vi "Test_Read_Dataset_From_Disk.vi"(8 "error in (no error)":errorcluster) -> (0 "error out":errorcluster)   [LabVIEW 2018]
doc: "This VI inits a waveform generation session for AWG-5421. This is a basic example that shows how to setup the board in order to generate waveforms according to a script. \nBy default this configuration uses one channel CH0, and one script trigger ScriptTrigger0. The ScriptTrigger0 is waiting for an external trigger : i.e. a digital Edge on pin PFI 0 by default.\n\nThere are various options for the script to be used. Consult the Script control help for more information on configuring the example for specific scripts."
uses:
  <vilib>/Analysis/NI_AALPro.lvlib
panel:
  in  "Cut Data ?":bool
  out "Mass Spectrum 2":cluster{"mass":sgl[], sgl[]}(graph)
  out "Mass Spectrum":cluster{"mass":sgl[], sgl[]}(graph)
  out "Signal 2":cluster{sgl[], sgl[]}(graph)
  out "df 2":dbl caption="df" format="%0.2f"
  out "Frequency Spectrum 2":cluster{dbl[], dbl[]}(graph)
  in  "End Signal":i32=200000
  in  "Start Signal":i32
  out "offset":sgl
  out "Frequency Spectrum":cluster{dbl[], "Power Spectrum (V^2 rms)":dbl[]}(graph)
  out "df":dbl format="%0.2f"
  out "Vertical Range in data":sgl
  out "Signal":cluster{sgl[], sgl[]}(graph)
  out "Time Step":sgl
  in  "chemin du fichier":path=path "D:/PIRENEA/DATA/2016/data_2016_11_22/2016_11_22_016.A00"
  out "Data Size (samples)":i32
  out "Total Size (bytes)":i64
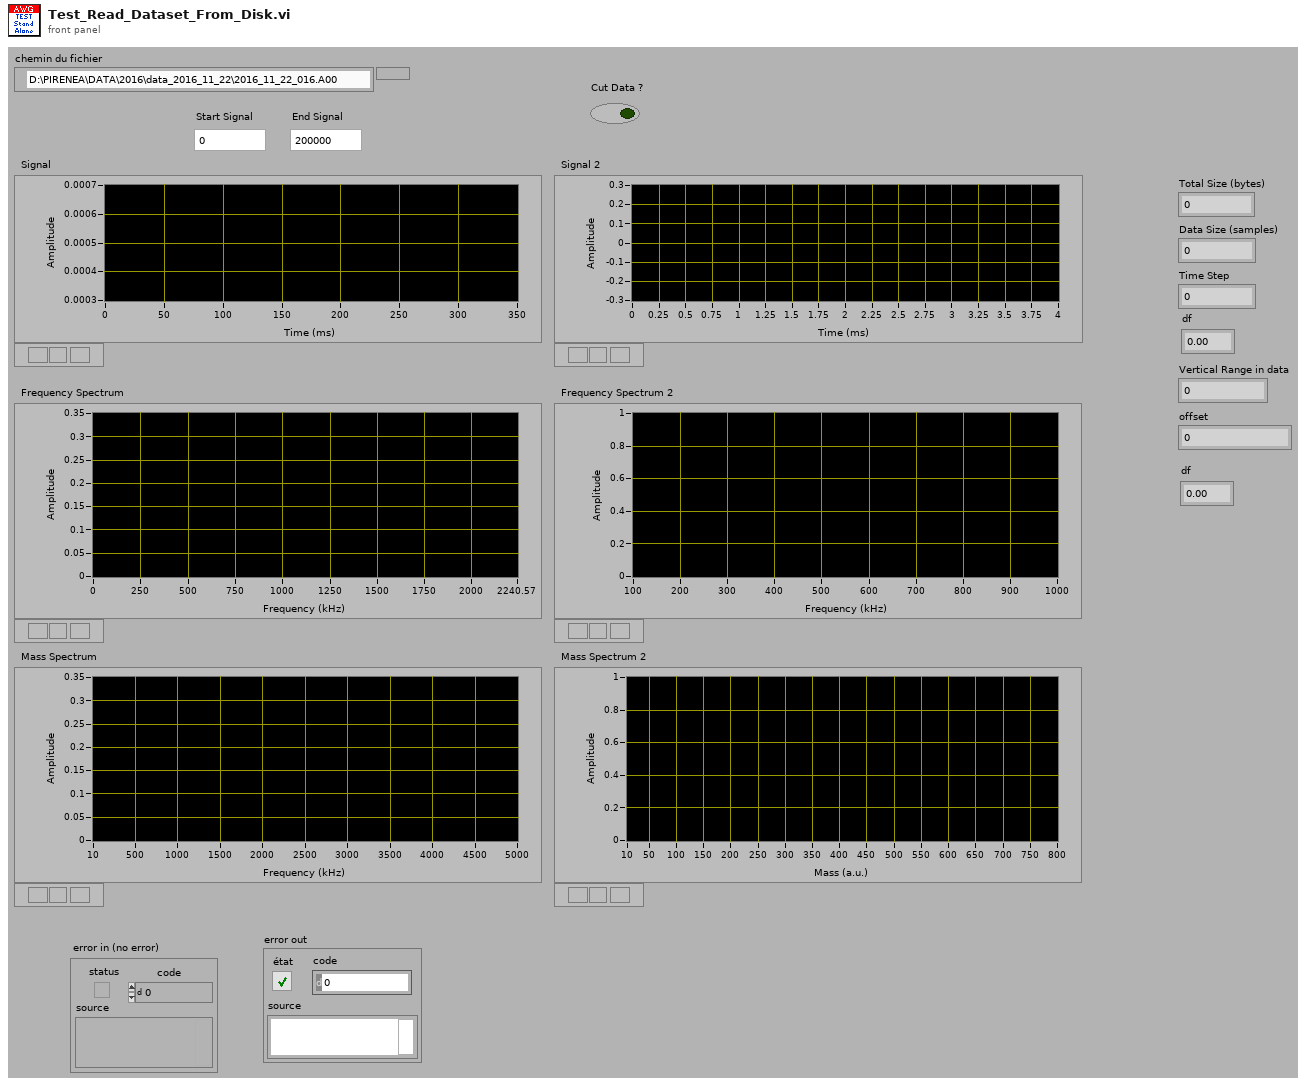
[diagram p1: front panel]
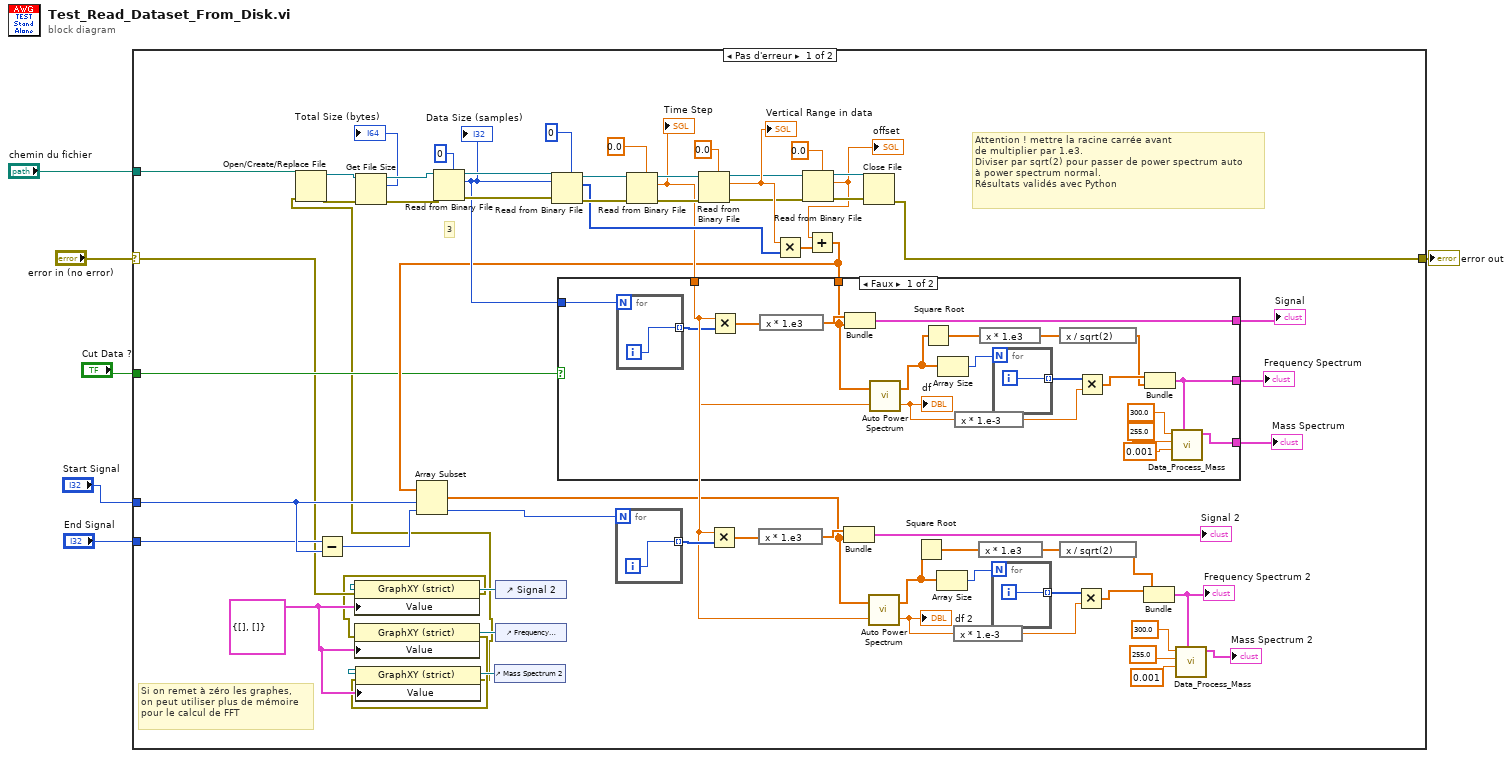
[diagram p0: block diagram]
diagram:
  n1 = case shown="Pas d'erreur" "error in (no error)" {
    selector: "error in (no error)" -> [w10 w95]
    tunnel: [w53 w95] -> w6
    tunnel: "chemin du fichier" -> [w60 _]
    tunnel: "Start Signal" -> [w24 _]
    tunnel: "End Signal" -> [w23 _]
    tunnel: "Cut Data ?" -> [w18 _]
    frame No Error {
      w11 = cluster{sgl[], sgl[]} {[], []} ("Valeur")
      # "Si on remet à zéro les graphes,\non peut utiliser plus de mémoire\npour le calcul de FFT"
      # "Attention ! mettre la racine carrée avant\nde multiplier par 1.e3.\nDiviser par sqrt(2) pour passer de power spectrum auto\nà power spectrum normal.\nRésultats validés avec Python"
      # "3"
      n2 = Subtract(x=w23, y=w24) -> (x-y=w32:i32)
      n3 = control-ref of="Mass Spectrum 2"() -> (w12:refnum<vi>)
      n4 = control-ref of="Signal 2"() -> (w14:refnum<vi>)
      n5 = property class="GraphXY (strict)"(reference=w14, error in=w10, "Value"=w11) -> (error out=w9:errorcluster)  [unwired: 1 out]
      n6 = control-ref of="Frequency Spectrum 2"() -> (w13:refnum<vi>)
      n7 = property class="GraphXY (strict)"(reference=w13, error in=w9, "Value"=w11) -> (error out=w8:errorcluster)  [unwired: 1 out]
      n8 = property class="GraphXY (strict)"(reference=w12, error in=w8, "Value"=w11) -> (error out=w7:errorcluster)  [unwired: 1 out]
      n9 = Open/Create/Replace File(file path (use dialog)=w60, error in=w7) -> (refnum out=w68:refnum<file>, error out=w67:errorcluster)  [unwired: 4 in, 1 out]
      n10 = Get File Size(file=w68, error in=w67) -> (refnum out=w66:refnum<file>, size (in bytes)=→"Total Size (bytes)":i64, 0:w65:errorcluster)
      n11 = Read from Binary File(5:0, 8:w65, 11:w66) -> (0:w62:errorcluster, 2:w51:i32, 3:w63:refnum<file>)  [unwired: 3 in, 1 out]
      "Data Size (samples)" <- w51
      n12 = Read from Binary File(5:i16 0, 8:w62, 10:w51, 11:w63) -> (0:w58:errorcluster, 2:w52:i16[], 3:w59:refnum<file>)  [unwired: 2 in, 1 out]
      n13 = for {
        N: w32 -> [_]
        tunnel: [w94] -> w33 mode=indexing
        i -> [w94]
      }
      n14 = Read from Binary File(5:sgl 0.0 ("type de données"), 8:w58, 11:w59) -> (0:w56:errorcluster, 2:w31:sgl, 3:w55:refnum<file>)  [unwired: 3 in, 1 out]
      "Time Step" <- w31
      n15 = Read from Binary File(5:sgl 0.0 ("type de données"), 8:w56, 11:w55) -> (0:w47:errorcluster, 2:w50:sgl, 3:w49:refnum<file>)  [unwired: 3 in, 1 out]
      "Vertical Range in data" <- w50
      n16 = Multiply(x=w31, y=w33) -> (x*y=w40:sgl[])
      n17 = expression code="x * 1.e3"(w40) -> (w41:sgl[])
      n18 = Multiply(x=w50, y=w52) -> (x*y=w44:sgl[])
      n19 = Read from Binary File(5:sgl 0.0, 8:w47, 11:w49) -> (0:w46:errorcluster, 2:w43:sgl, 3:w48:refnum<file>)  [unwired: 3 in, 1 out]
      "offset" <- w43
      n20 = Add(x=w43, y=w44) -> (x+y=w19:sgl[])
      n21 = Array Subset(array=w19, index=w24, length=w32) -> (w30:sgl[])
      n22 = case shown="Faux" w18 {
        tunnel: w51 -> [w90 _]
        tunnel: w31 -> [w79 _]
        tunnel: w19 -> [w73 _]
        tunnel: [w72 _] -> w17
        tunnel: [w71 _] -> w16
        tunnel: [w70 _] -> w15
        frame False {
          n23 = for {
            N: w90 -> [_]
            tunnel: [w92] -> w89 mode=indexing
            i -> [w92]
          }
          n24 = Multiply(x=w79, y=w89) -> (x*y=w83:sgl[])
          n25 = expression code="x * 1.e3"(w83) -> (w82:sgl[])
          n26 = Bundle(w82, w73) -> (w72:cluster{sgl[], sgl[]})  [unwired: 1 in]
          n27 = call <vilib>:"Auto Power Spectrum.vi"("dt"=w79, "Signal (V)"=w73) -> ("df"=w85:dbl, "Power Spectrum (V^2 rms)"=w81:dbl[])
          "df" <- w85
          n28 = Square Root(x=w81) -> (sqrt(x)=w75:dbl[])
          n29 = Array Size(array=w81) -> (size(s)=w88:i32)
          n30 = expression code="x * 1.e-3"(w85) -> (w84:dbl)
          n31 = expression code="x * 1.e3"(w75) -> (w80:dbl[])
          n32 = for {
            N: w88 -> [_]
            tunnel: [w91] -> w87 mode=indexing
            i -> [w91]
          }
          n33 = expression code="x / sqrt(2)"(w80) -> (w74:dbl[])
          n34 = Multiply(x=w87, y=w84) -> (x*y=w86:dbl[])
          n35 = Bundle(w86, w74) -> (w71:cluster{dbl[], dbl[]})  [unwired: 1 in]
          n36 = call "Data_Process_Mass.vi"("Frequency Spectrum"=w71, "Mag. Frequency (kHz)"=0.001, "Cycl. Frequency (kHz)"=255.0, "Reference mass (u)"=300.0) -> ("Mass Spectrum"=w70:cluster{"mass":sgl[], sgl[]})  [unwired: 6 in, 1 out]
        }
        frame True {
        }
      }
      "Signal" <- w17
      "Frequency Spectrum" <- w16
      "Mass Spectrum" <- w15
      n37 = Bundle(w41, w30) -> (→"Signal 2":cluster{sgl[], sgl[]})  [unwired: 1 in]
      n38 = Close File(refnum=w48, error in=w46) -> (error out=w53:errorcluster)  [unwired: 1 out]
      n39 = call <vilib>:"Auto Power Spectrum.vi"("dt"=w31, "Signal (V)"=w30) -> ("df"=w38:dbl, "Power Spectrum (V^2 rms)"=w42:dbl[])
      "df 2" <- w38
      n40 = Square Root(x=w42) -> (sqrt(x)=w22:dbl[])
      n41 = Array Size(array=w42) -> (size(s)=w35:i32)
      n42 = expression code="x * 1.e-3"(w38) -> (w39:dbl)
      n43 = expression code="x * 1.e3"(w22) -> (w29:dbl[])
      n44 = for {
        N: w35 -> [_]
        tunnel: [w93] -> w36 mode=indexing
        i -> [w93]
      }
      n45 = expression code="x / sqrt(2)"(w29) -> (w21:dbl[])
      n46 = Multiply(x=w36, y=w39) -> (x*y=w37:dbl[])
      n47 = Bundle(w37, w21) -> (w25:cluster{dbl[], dbl[]})  [unwired: 1 in]
      "Frequency Spectrum 2" <- w25
      n48 = call "Data_Process_Mass.vi"("Frequency Spectrum"=w25, "Mag. Frequency (kHz)"=0.001, "Cycl. Frequency (kHz)"=255.0, "Reference mass (u)"=300.0) -> ("Mass Spectrum"=→"Mass Spectrum 2":cluster{"mass":sgl[], sgl[]})  [unwired: 6 in, 1 out]
    }
    frame Error {
    }
  }
  "error out" <- w6
